vi "uTransport_SendMsg Core.vi"(8 "error in (no error)":errorcluster, 10 "Msg":refnum<class "uMsg.lvclass">, 11 "uTransport_uActor in":refnum<class "uTransport_uActor.lvclass">) -> (0 "error out":errorcluster, 3 "uTransport_uActor out":refnum<class "uTransport_uActor.lvclass">)   [LabVIEW 2023, in "uLib.lvlib" / "uTransport_uActor.lvclass"]
uses:
  uTransport_uActor.lvclass
  uMsg/uMsg/uMsg.lvclass
  uTransport_uActor.lvclass/uTransport_uActor.ctl
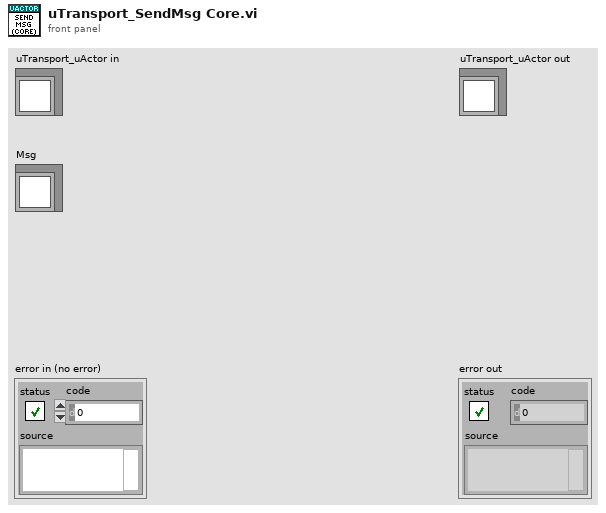
[diagram p1: front panel]
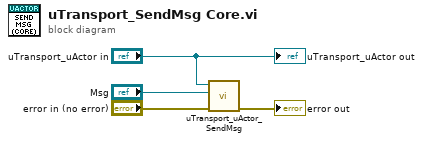
[diagram p0: block diagram]
diagram:
  n1 = call "uTransport_uActor_SendMsg.vi"("error in (no error)"="error in (no error)", "Msg"="Msg", "uTransport_uActor in"="uTransport_uActor in") -> ("error out"=→"error out":errorcluster)  [unwired: 8 in]
  "uTransport_uActor out" <- "uTransport_uActor in"
